vi "runLoadHTSocketLog.vi"() -> ()   [LabVIEW 2012]
uses:
  <vilib>/Utility/file.llb/Read From Spreadsheet File (string).vi
  <vilib>/regexp/Match Regular Expression.xnode
panel:
  in  "file (use dialog)":path=path "C:/temp/ht/Socket/SocketLog.txt"
  out "concatenated string 2":string
  in  "file path (dialog if empty)":path=path "C:/temp/ht/now/HTentity.txt"
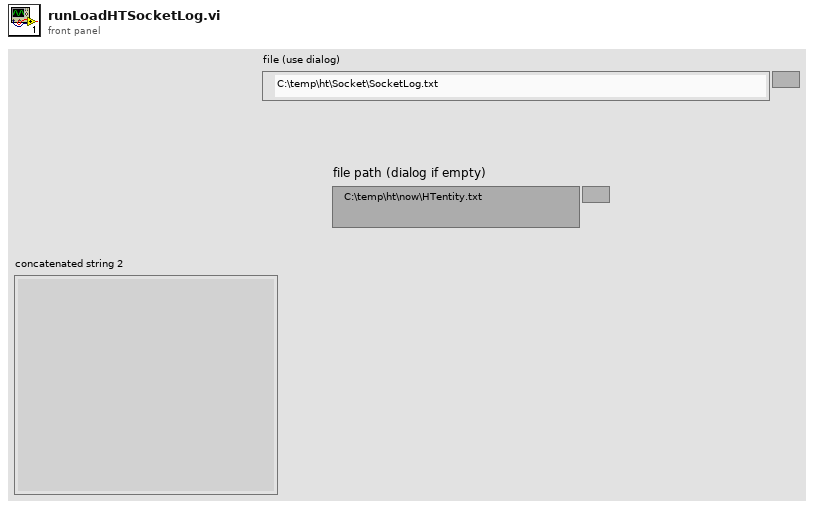
[diagram p1: front panel]
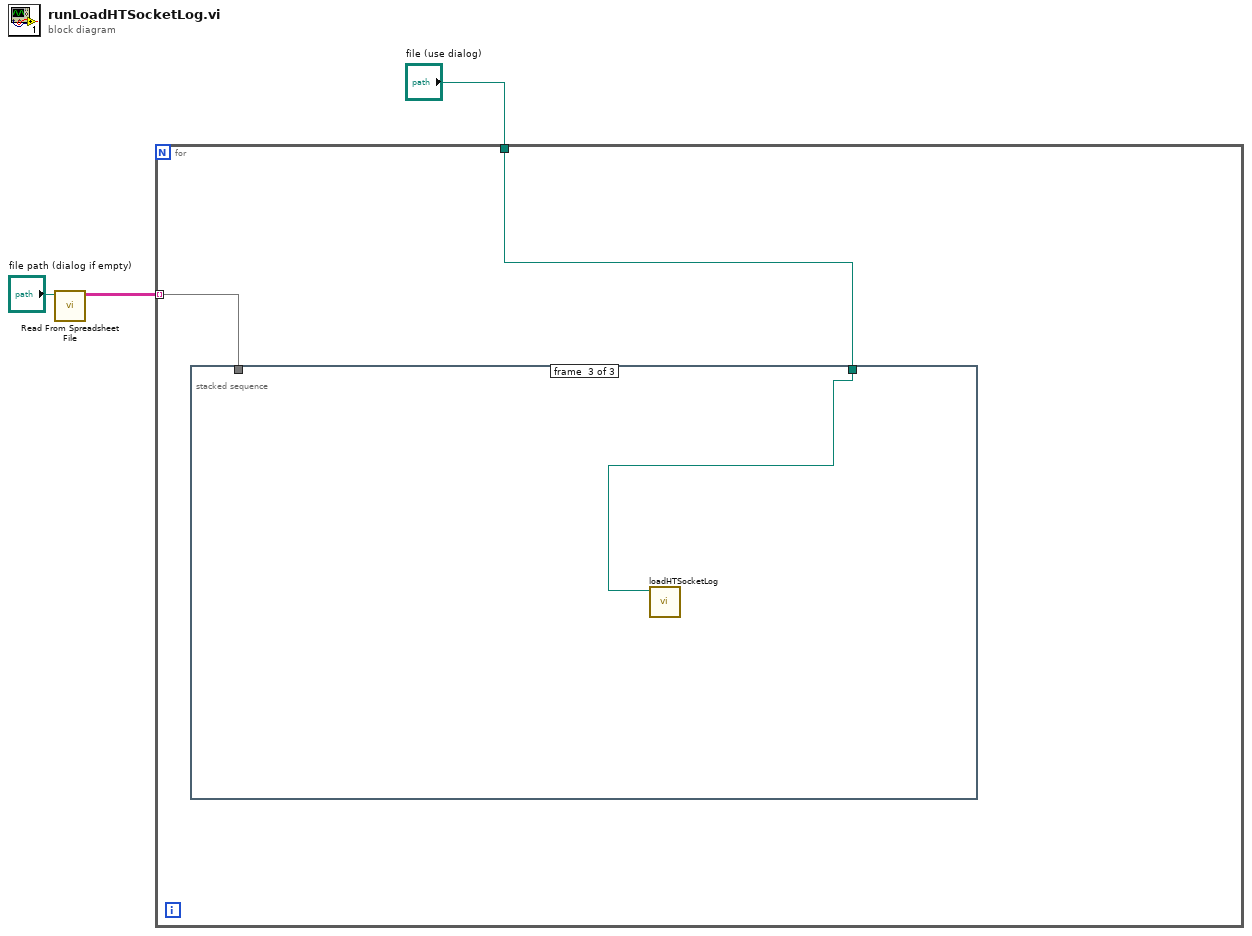
[diagram p0: block diagram]
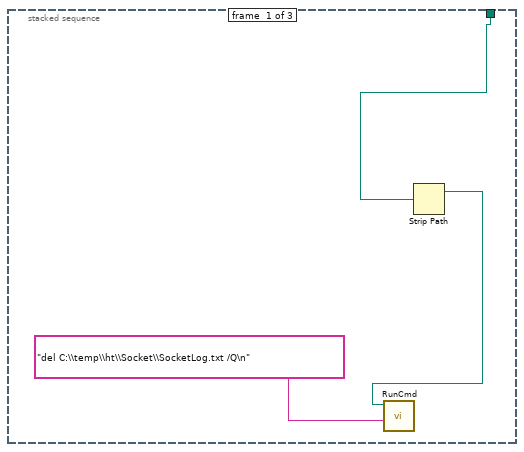
[diagram p2: hidden frame]
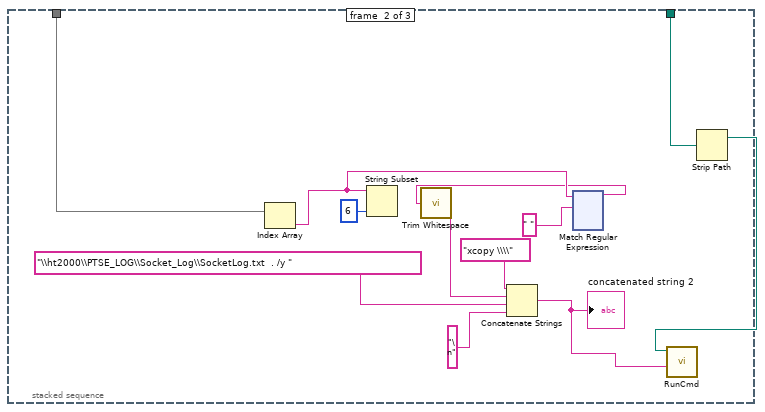
[diagram p3: hidden frame]
diagram:
  n1 = call-poly <vilib>:"Read From Spreadsheet File.vi"("file path (dialog if empty)"="file path (dialog if empty)") -> ("all rows"=w2:string[][])  [unwired: 6 in, 4 out]
  n2 = for {
    tunnel: w2 -> [w5] mode=indexing
    tunnel: "file (use dialog)" -> [w4]
    n3 = stacked-sequence {
      tunnel: w5 -> [_ w11 _]
      tunnel: w4 -> [w6 w10 w132]
      frame #0 {
        n4 = Strip Path(path=w6) -> (stripped path=w8:path)  [unwired: 1 out]
        n5 = call "RunCmd.vi"("Cmd String"="del C:\\temp\\ht\\Socket\\SocketLog.txt /Q\n", "working directory"=w8) -> ()  [unwired: 8 in, 2 out]
      }
      frame #1 {
        n6 = Index Array(array=w11) -> (element=w16:string)  [unwired: 1 in]
        n7 = String Subset(string=w16, length (rest)=6 ("length (rest)")) -> ()  [unwired: 1 in, 1 out]
        n8 = xnode "Match Regular Expression"("input string"=w16, "regular expression"=" ") -> ("before match"=w15:string)  [unwired: 4 in, 4 out]
        n9 = call <vilib>:"Trim Whitespace.vi"("string"=w15) -> ("trimmed string"=w12:string)  [unwired: 1 in]
        n10 = Concatenate Strings("xcopy \\\\" ("string"), w12, "\\ht2000\\PTSE_LOG\\Socket_Log\\SocketLog.txt  . /y " ("string"), "\n" ("string")) -> (w19:string)
        "concatenated string 2" <- w19
        n11 = Strip Path(path=w10) -> (stripped path=w9:path)  [unwired: 1 out]
        n12 = call "RunCmd.vi"("Cmd String"=w19, "working directory"=w9) -> ()  [unwired: 8 in, 2 out]
      }
      frame #2 {
        n13 = call "loadHTSocketLog.vi"("file (use dialog)"=w132) -> ()  [unwired: 11 in]
      }
    }
  }
